vi "network-ping.vi"(8 "error in (no error)":errorcluster, 11 "ip_address in":string) -> (0 "error out":errorcluster, 1 "% loss":i32, 2 "ping_success?":bool, 3 "ip_address out":string)   [LabVIEW 2015, in "lv-bin-windows.lvlib" / "v1.lvlib"]
uses:
  v1.lvlib
  <userlib>/antonio-alexander/lv-bin/lv-bin/public/api/v1/v1.lvlib
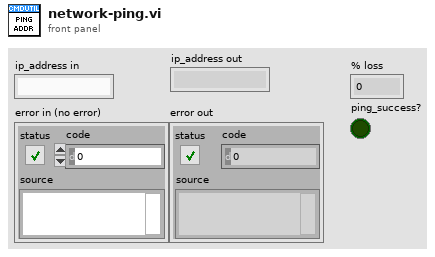
[diagram p1: front panel]
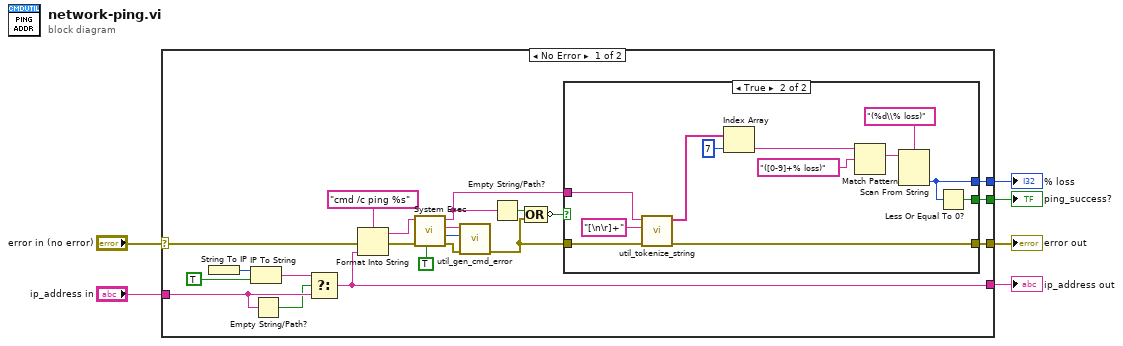
[diagram p0: block diagram]
diagram:
  n1 = case shown="No Error" "error in (no error)" {
    selector: "error in (no error)" -> [w19 w41]
    tunnel: "ip_address in" -> [w21 _]
    tunnel: [w18 _] -> w4
    tunnel: [w17 _] -> w3
    tunnel: [w9 w41] -> w2
    tunnel: [w12 _] -> w1
    frame No Error {
      n2 = String To IP() -> (0:w16:u32)  [unwired: 1 in]
      n3 = IP To String(1:TRUE ("dot notation? (F)"), 2:w16) -> (0:w22:string)
      n4 = Empty String/Path?(string/path=w21) -> (empty?=w20:bool)
      n5 = Select(t=w22, s=w20, f=w21) -> (s? t:f=w12:string)
      n6 = Format Into String(format string="cmd /c ping %s", error in=w19, w12) -> (resulting string=w26:string, error out=w25:errorcluster)  [unwired: 1 in]
      n7 = call <vilib>:"System Exec.vi"("run minimized? (F)"=TRUE, "error in (no error)"=w25, "command line"=w26) -> ("error out"=w11:errorcluster, "return code"=w7:i32, "standard error"=w8:string, "standard output"=w15:string)  [unwired: 5 in]
      n8 = call <userlib>:"util_gen_cmd_error.vi"("error in (no error)"=w11, "return_code"=w7, "standard_error"=w8) -> ("error out"=w10:errorcluster)  [unwired: 8 in]
      n9 = Empty String/Path?(string/path=w15) -> (empty?=w14:bool)
      n10 = Compound Arithmetic op=OR(w14, w10) -> (invert w13:bool)
      n11 = case shown="True" w13 {
        tunnel: [_ w36] -> w18
        tunnel: [_ w35] -> w17
        tunnel: w15 -> [_ w34]
        tunnel: w10 -> [w28 w31]
        tunnel: [w28 w30] -> w9
        frame False {
        }
        frame True {
          n12 = call <userlib>:"util_tokenize_string.vi"("error in (no error)"=w31, "delimiter"="[\n\r]+" ("delimiter ([\\s\\t\\n\\r]+)"), "input_string"=w34) -> ("error out"=w30:errorcluster, "before_match []"=w33:string[])  [unwired: 6 in, 1 out]
          n13 = Index Array(array=w33, index=7) -> (element=w40:string)
          n14 = Match Pattern(string=w40, regular expression="([0-9]+% loss)") -> (match substring=w38:string)  [unwired: 1 in, 3 out]
          n15 = Scan From String(format string="(%d\\% loss)", input string=w38) -> (output 1=w35:i32)  [unwired: 3 in, 3 out]
          n16 = Less Or Equal To 0?(x=w35) -> (x <= 0?=w36:bool)
        }
      }
    }
    frame Error {
    }
  }
  "error out" <- w2
  "ping_success?" <- w4
  "% loss" <- w3
  "ip_address out" <- w1
